vi "PID Motors.vi"(3 "stop":bool, 4 "Speed B":dbl(slide)=-0.016713091922005565 scale=-2.0..2.0, 5 "Speed A":dbl(slide)=-0.016713091922005565 scale=-2.0..2.0) -> (1 "PID B":cluster{"Setpoint":dbl, "dx/dt":dbl}(graph), 2 "PID A":cluster{"Setpoint":dbl, "dx/dt":dbl}(graph))   [LabVIEW 2017]
uses:
  <vilib>/myRIO/Common/Instrument Driver Framework/myRIO v1.0/UART/vis/myRIO v1.0 Close UART.vi
  <vilib>/myRIO/Common/Instrument Driver Framework/Utilities/vis/FPGA Ref Manager.vi
  <vilib>/myRIO/Common/Instrument Driver Framework/myRIO v1.0/myRIO v1.0 Reset FPGA.vi
  <vilib>/myRIO/Common/Instrument Driver Framework/myRIO v1.0/IRQ/vis/myRIO v1.0 IRQ Info FGV.vi
  <vilib>/myRIO/Common/Instrument Driver Framework/myRIO v1.0/IRQ/vis/myRIO v1.0 Timer IRQ Info FGV.vi
  <vilib>/myRIO/Common/Instrument Driver Framework/myRIO v1.0/IRQ/vis/myRIO v1.0 ISR Agent.vi
  <vilib>/myRIO/Instrument Drivers/Utilities/Utilities.lvlib
panel:
  in  "PID gains":T1={"proportional gain (Kc)"=0.015, "integral time (Ti, min)"=0.003, "derivative time (Td, min)"=0.0} {"derivative time (Td, min)" format="%.6f"; "integral time (Ti, min)" format="%.6f"; "proportional gain (Kc)" format="%.6f"}
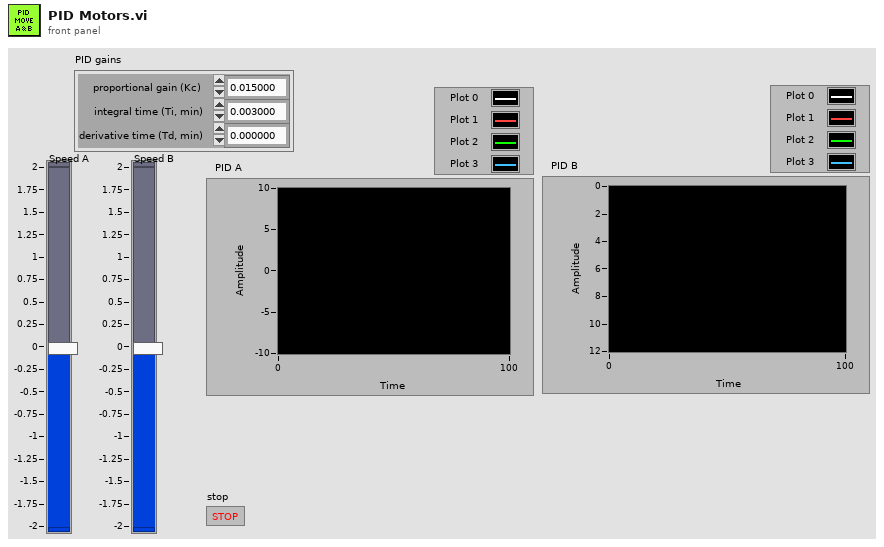
[diagram p1: front panel]
types:
  T1 = cluster{"proportional gain (Kc)":dbl, "integral time (Ti, min)":dbl, "derivative time (Td, min)":dbl}
  T2 = cluster{"Setpoint":dbl, "output":dbl, "dx/dt":dbl}
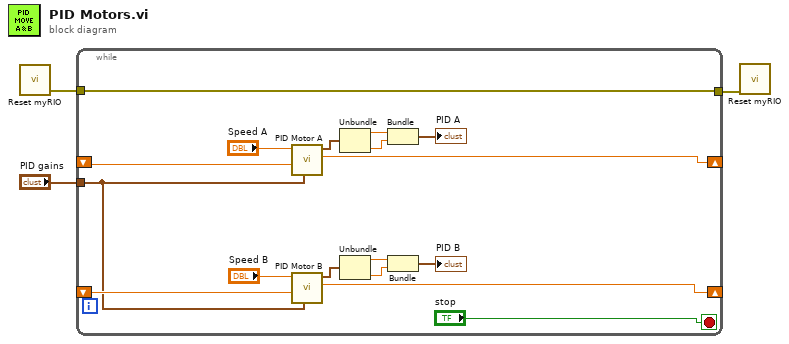
[diagram p0: block diagram]
diagram:
  n1 = call <vilib>:"Reset myRIO.vi"() -> ("error out"=w3:errorcluster)  [unwired: 11 in]
  n2 = while {
    shift-right: [w18] -> _
    shift-left: _ -> [w16]
    tunnel: [w19] -> w2
    tunnel: w3 -> [w19]
    shift-right: [w17] -> _
    shift-left: _ -> [w15]
    tunnel: "PID gains" -> [w14]
    stop <- "stop" stop-if-true
    n3 = call "PID Motor A.vi"("PID gains"=w14, "input"=w16, "Setpoint A0"="Speed A") -> ("output"=w18:dbl, "Speed A0"=w12:T2)  [unwired: 3 in, 4 out]
    n4 = call "PID Motor B.vi"("PID gains"=w14, "input"=w15, "Setpoint B0"="Speed B") -> ("output"=w17:dbl, "Speed B0"=w13:T2)  [unwired: 3 in, 4 out]
    n5 = Unbundle(w12) -> ("Setpoint"=w11:dbl, "dx/dt"=w10:dbl)  [unwired: 1 out]
    n6 = Unbundle(w13) -> ("Setpoint"=w9:dbl, "dx/dt"=w8:dbl)  [unwired: 1 out]
    n7 = Bundle("Setpoint"=w11, "dx/dt"=w10) -> (→"PID A":cluster{"Setpoint":dbl, "dx/dt":dbl})  [unwired: 1 in]
    n8 = Bundle("Setpoint"=w9, "dx/dt"=w8) -> (→"PID B":cluster{"Setpoint":dbl, "dx/dt":dbl})  [unwired: 1 in]
  }
  n9 = call <vilib>:"Reset myRIO.vi"("error in (no error)"=w2) -> ()  [unwired: 10 in, 1 out]
